vi "rs3 Advanced set SLO Penalty3.vi"(8 "error in (no error)":errorcluster, 10 "ST SLO Penalty":T1, 11 "device in":u64) -> (0 "error out":errorcluster, 1 "error":u64, 3 "Dev out":u64)   [LabVIEW 2018, in "libRealSense3.lvlib"]
doc: "Opens communication to a specific RealSense Device."
uses:
  libRealSense3.lvlib
  realsense2.dll
panel:
  # "RS3 Adv. Set SLO Penalty 2"
  # "(C) 2017 Intel Corp.,  AGJ"
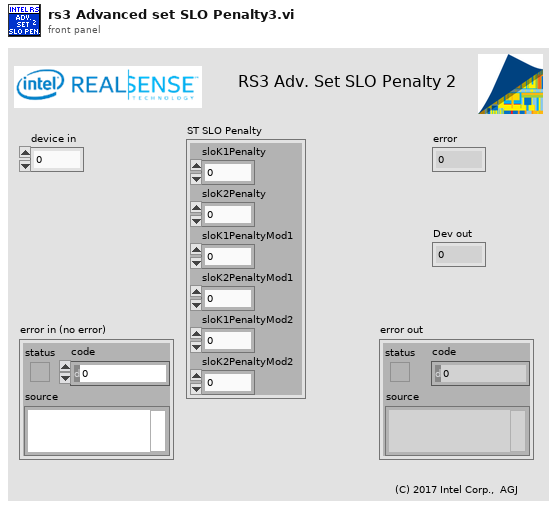
[diagram p1: front panel]
types:
  T1 = cluster{"sloK1Penalty":u32, "sloK2Penalty":u32, "sloK1PenaltyMod1":u32, "sloK2PenaltyMod1":u32, "sloK1PenaltyMod2":u32, "sloK2PenaltyMod2":u32}
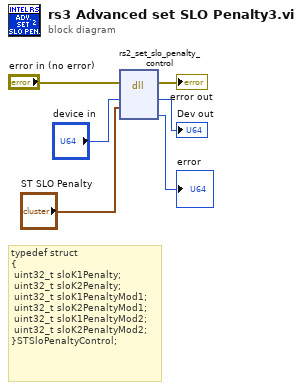
[diagram p0: block diagram]
diagram:
  # "typedef struct\n{\n\tuint32_t sloK1Penalty;\n\tuint32_t sloK2Penalty;\n\tuint32_t sloK1PenaltyMod1;\n\tuint32_t sloK2PenaltyMod1;\n\tuint32_t sloK1PenaltyMod2;\n\tuint32_t sloK2PenaltyMod2;\n}STSloPenaltyControl;"
  n1 = dll-call lib="C:/Users/aaron.jencks/Documents/GitHub/emerson_seed_object_detection/LabVIEW/Projects/Paul's Video Viewer/Classes/Realsense Cam/realsense_wrapper_api/realsense2.dll" fn="rs2_set_slo_penalty_control"(error in="error in (no error)", "device"="device in", "ST SLO Penalty"="ST SLO Penalty") -> (error out=→"error out":errorcluster, "device"=→"Dev out":u64, "error"=→"error":u64)  [unwired: 5 in, 1 out]
